vi "LVProjectShortcut_CreateNewWizard_Finalize.vi"(10 "Item":T1, 11 "Wizard":T1) -> ()   [LabVIEW 2017]
doc: "NI Confidential \n\n/**\n@brief This VI is called by the framework when an item of this type is first created.\n\n@author Joel Dixon\n\n@par Sample_Item_Init.vi\n This VI might typically set the popup menu for this item by calling mxLvSetPopupMenu.vi, set the icon for the item by calling mxLvSetIcon.vi, and set a name to be displayed in the tree by calling mxLvSetName.vi. \n\n@param \"Object\" [in] \nPassed by the framework as a reference to 'this' item in the tree. This parameter can be passed as the 'item' parameter for any of the mxLv** VIs, such as mxLvCreateItems.vi.\n*/"
uses:
  <resource>/Framework/Providers/API/ItemRef.ctl
  <resource>/Framework/Providers/API/mxLvUpdateUI.ctl
  <resource>/Framework/Providers/API/mxLvSetStringProperty.vi
  <resource>/Framework/Providers/API/mxLvSetBooleanProperty.vi
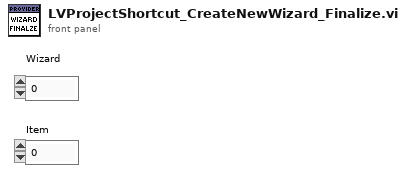
[diagram p1: front panel]
types:
  T1 = typedef "ItemRef.ctl" = u64
  T2 = typedef "mxLvUpdateUI.ctl" = cluster{"Action":u32, "Optional param 1":string, "Optional param 2":i32, "Optional param 3":string}
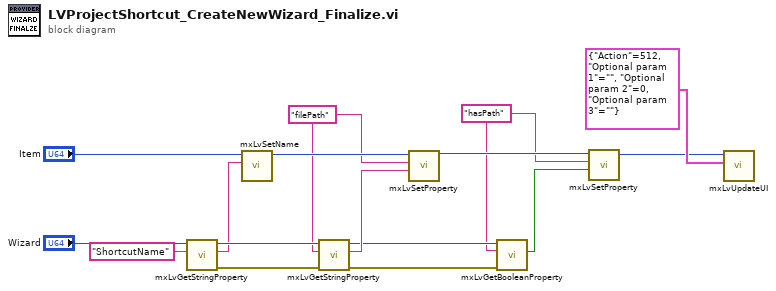
[diagram p0: block diagram]
diagram:
  w3 = "hasPath" ("Tag")
  w10 = "filePath" ("Tag")
  n1 = call <resource>:"mxLvGetStringProperty.vi"("Tag"="ShortcutName", "Item"="Wizard") -> ("Error Out"=w6:errorcluster, "Value"=w8:string, "Item"=w12:T1)  [unwired: 7 in]
  n2 = call <resource>:"mxLvSetName.vi"("Name"=w8, "Item"="Item") -> ("Item"=w11:T1)  [unwired: 8 in, 1 out]
  n3 = call <resource>:"mxLvGetStringProperty.vi"("Error In"=w6, "Tag"=w10, "Item"=w12) -> ("Error Out"=w4:errorcluster, "Value"=w9:string, "Item"=w5:T1)  [unwired: 6 in]
  n4 = call-poly <resource>:"mxLvSetProperty.vi"("Value (\"\")"=w9, "Tag"=w10, "Item"=w11) -> ("Item"=w7:T1)  [unwired: 7 in, 1 out]
  n5 = call <resource>:"mxLvGetBooleanProperty.vi"("error in"=w4, "Tag"=w3, "Item"=w5) -> ("Value"=w2:bool)  [unwired: 6 in, 2 out]
  n6 = call-poly <resource>:"mxLvSetProperty.vi"("Value (F)"=w2, "Tag"=w3, "Item"=w7) -> ("Item"=w1:T1)  [unwired: 7 in, 1 out]
  n7 = call <resource>:"mxLvUpdateUI.vi"("Update UI Settings"=T2 {"Action"=512, "Optional param 1"="", "Optional param 2"=0, "Optional param 3"=""}, "Item"=w1) -> ()  [unwired: 8 in, 2 out]
